vi "SP Update PF Indicator.vi"(5 "Parameters Measured":T9[](array[typedef]) {"Channel" min=1 max=99 step=1; "Parameter"."Stimulus Port" min=1 step=1; "Parameter"."Response Port" min=1 step=1}, 6 "References":T12, 7 "Pass? (f)":bool, 8 "Wait? (f)":bool, 9 "Filter Parameter":refnum<vi>, 10 "Limit Results":T1[](array[typedef]) {"Parameter"."Stimulus Port" min=1 step=1; "Parameter"."Response Port" min=1 step=1}, 11 "error in (no error)":errorcluster) -> (1 "Status Text":string, 3 "error out":errorcluster)   [LabVIEW 2011]
uses:
  TypeDefs/SP Parameter to Measure.ctl
  TypeDefs/SP Parameter.ctl
  TypeDefs/SP Calibration State.ctl
  TypeDefs/SP Measurement Format.ctl
  TypeDefs/SP Limit Results.ctl
  TypeDefs/SP Bandwidth Limit Results.ctl
  TypeDefs/SP Frequency Units.ctl
  TypeDefs/SP Ripple Limit Results.ctl
  TypeDefs/SP Format.ctl
  TypeDefs/SP Attenuation Limit Results.ctl
  TypeDefs/SP Skirt Limit Results.ctl
  <vilib>/Utility/miscctls.llb/LVRowAndColumnTypeDef.ctl
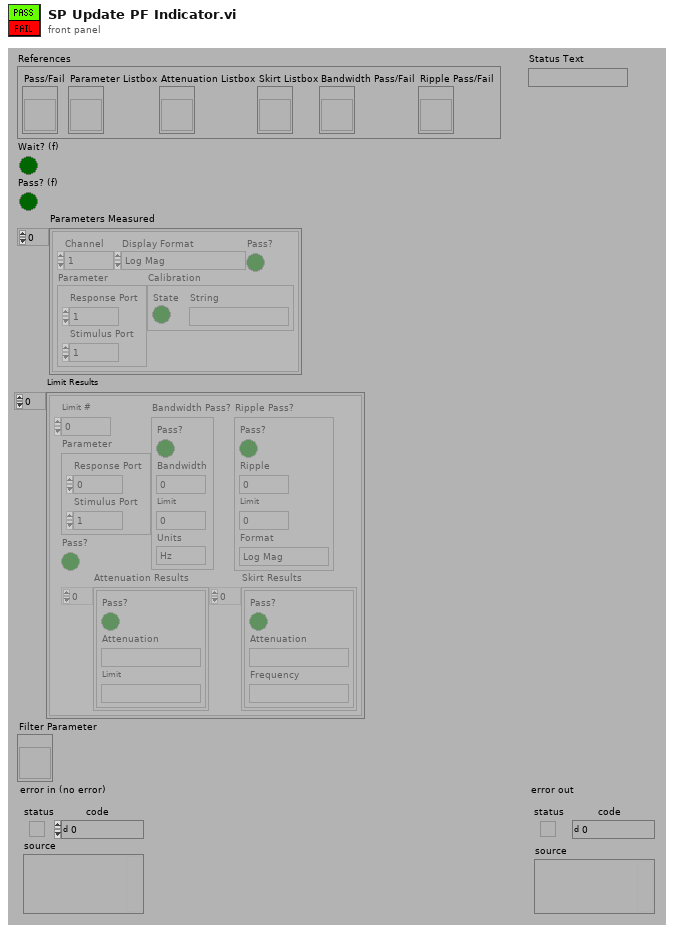
[diagram p1: front panel]
types:
  T1 = typedef "SP Limit Results.ctl" = cluster{"Limit #":i8, "Parameter":T2, "Bandwidth Pass?":T3, "Ripple Pass?":T5, "Attenuation Results":T7[], "Skirt Results":T8[], "Pass?":bool}
  T2 = typedef "SP Parameter.ctl" = cluster{"Stimulus Port":i8, "Response Port":i8}
  T3 = typedef "SP Bandwidth Limit Results.ctl" = cluster{"Pass?":bool, "Bandwidth":dbl, "Limit":dbl, "Units":T4}
  T4 = typedef "SP Frequency Units.ctl" = enum16{"Hz", "kHz", "MHz", "GHz", "Points"}
  T5 = typedef "SP Ripple Limit Results.ctl" = cluster{"Pass?":bool, "Ripple":dbl, "Limit":dbl, "Format":T6}
  T6 = typedef "SP Format.ctl" = enum16{"Log Mag", "Lin Mag", "SWR", "Phase", "Expanded Phase", "Delay", "Insertion Loss", "Isolation", "Return Loss"}
  T7 = typedef "SP Attenuation Limit Results.ctl" = cluster{"Pass?":bool, "Attenuation":string, "Limit":string}
  T8 = typedef "SP Skirt Limit Results.ctl" = cluster{"Pass?":bool, "Attenuation":string, "Frequency":string}
  T9 = typedef "SP Parameter to Measure.ctl" = cluster{"Channel":i8, "Parameter":T2, "Calibration":T10, "Display Format":T11, "Pass?":bool}
  T10 = typedef "SP Calibration State.ctl" = cluster{"State":bool, "String":string}
  T11 = typedef "SP Measurement Format.ctl" = enum32{"Log Mag", "Phase", "Delay", "Smith (R+jX)", "Polar (Re/Im)", "Linear Mag", "SWR", "Real", "Imaginary", "Smith (Lin/Phase)", "Smith (Log/Phase)", "Smith (Real/Imag)", "Smith (G+jB)", "Polar (Lin/Phase)", "Polar (Log/Phase)", "Expanded Phase", "Positive Phase", "Inverted Smith", "Unwrapped Phase", "Power Out", "Power In", "Linear Mag/Phase", "Log Mag/Phase", "Real/Imaginary"}
  T12 = cluster{"Pass/Fail":refnum<vi>, "Parameter Listbox":refnum<vi>, "Attenuation Listbox":refnum<vi>, "Skirt Listbox":refnum<vi>, "Bandwidth Pass/Fail":refnum<vi>, "Ripple Pass/Fail":refnum<vi>}
  T13 = typedef "LVRowAndColumnTypeDef.ctl" = cluster{"Row":i32, "Column":i32}
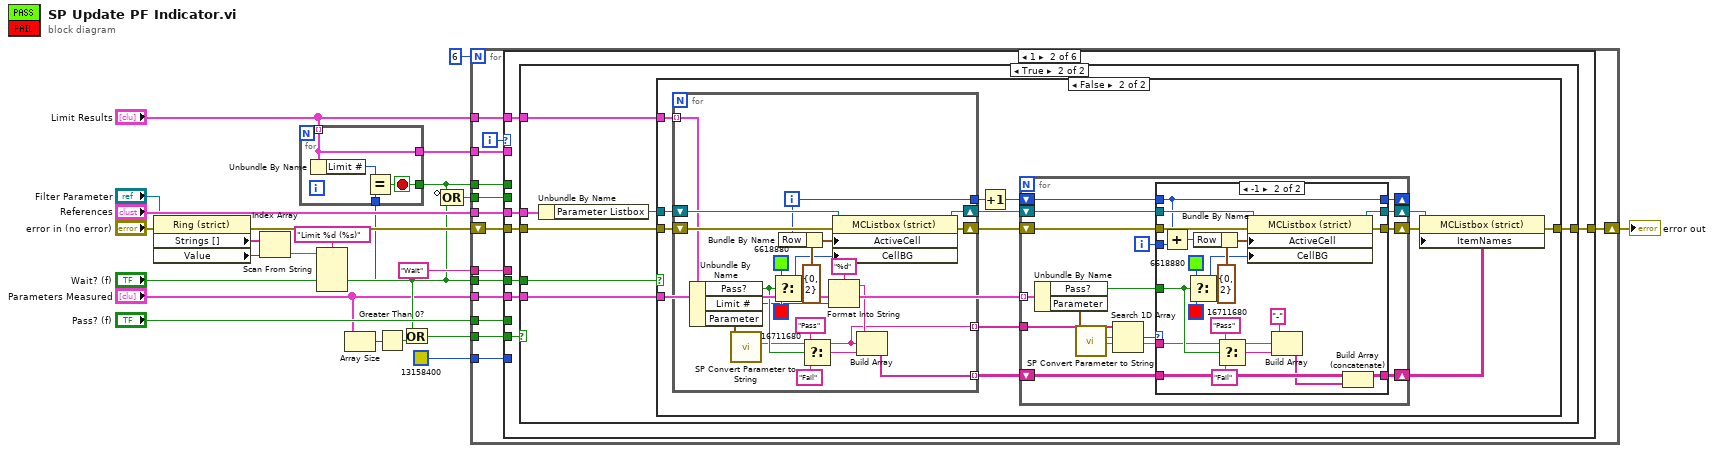
[diagram p0: block diagram]
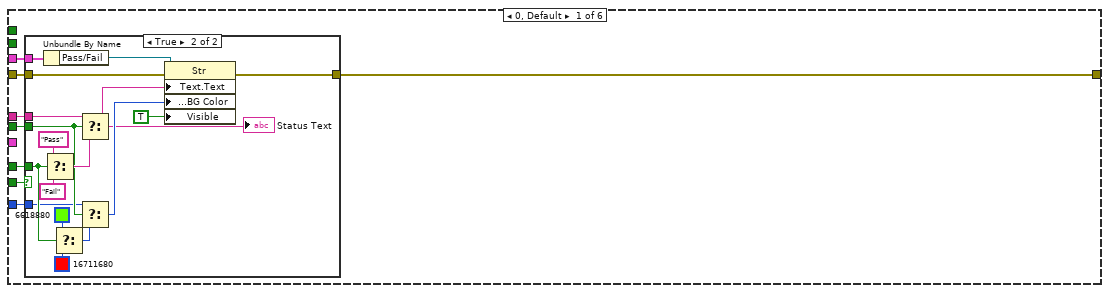
[diagram p2: hidden frame]
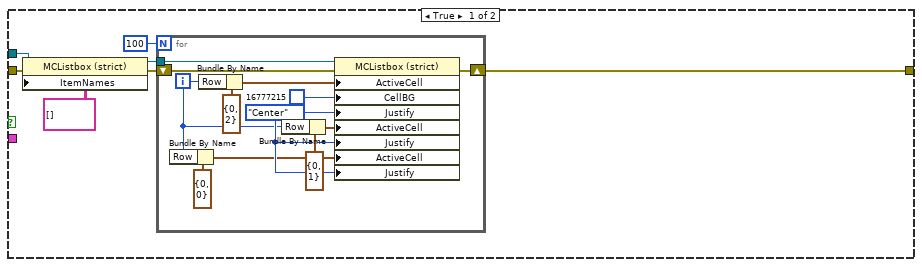
[diagram p5: hidden frame]
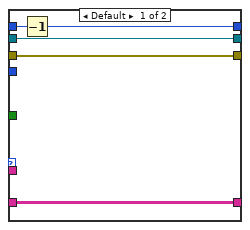
[diagram p6: hidden frame]
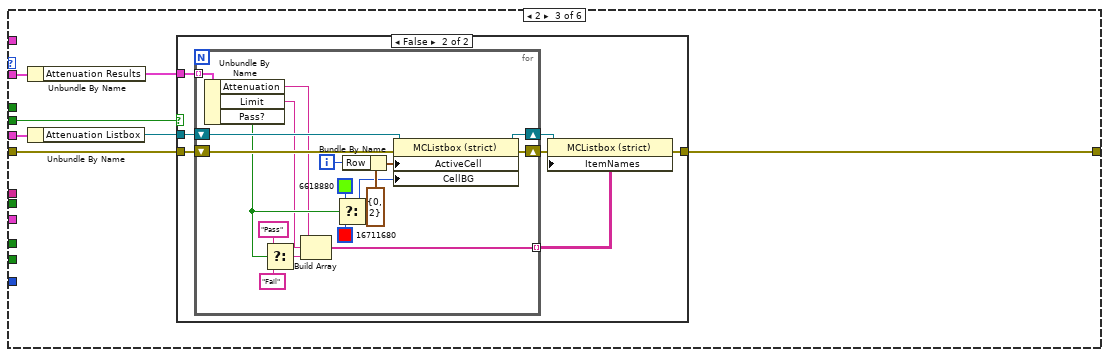
[diagram p7: hidden frame]
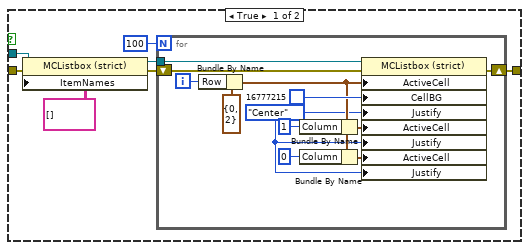
[diagram p8: hidden frame]
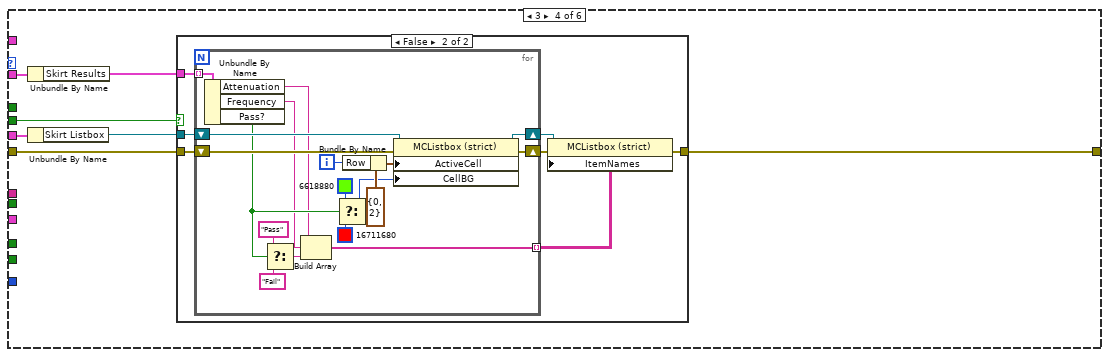
[diagram p9: hidden frame]
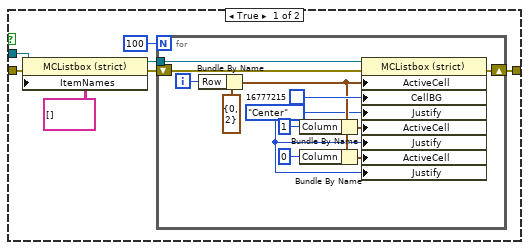
[diagram p10: hidden frame]
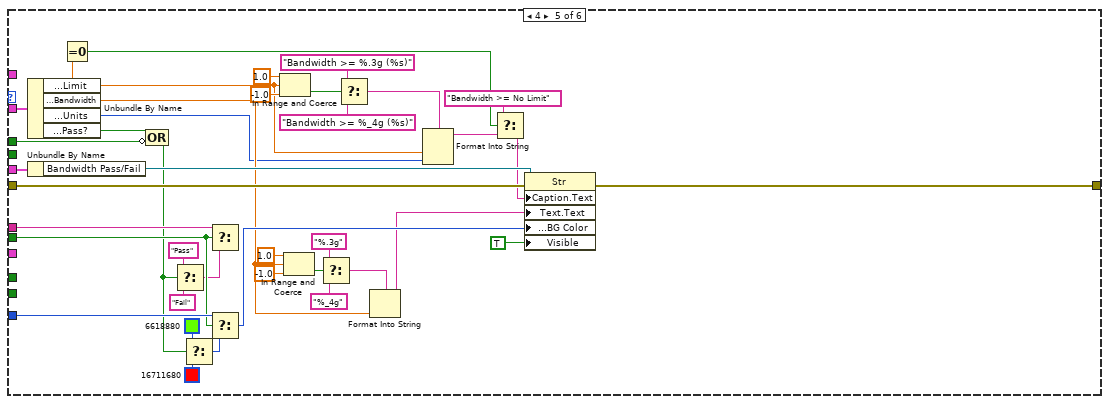
[diagram p11: hidden frame]
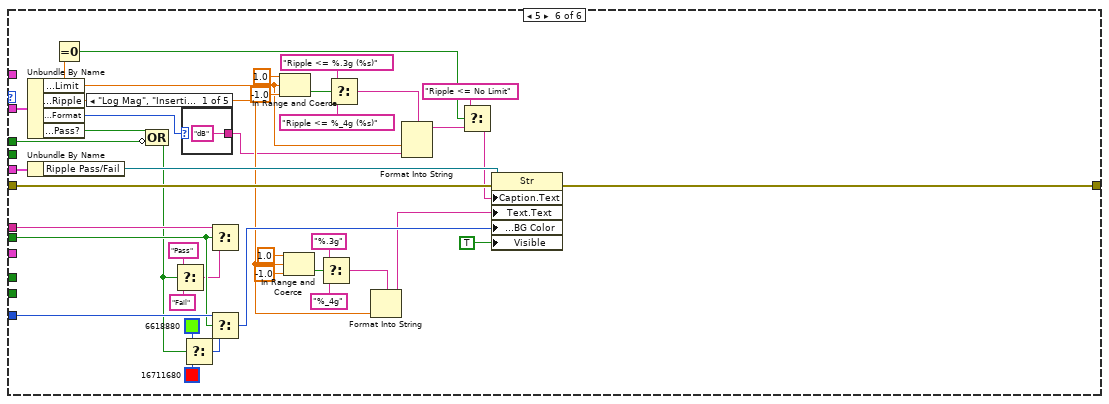
[diagram p12: hidden frame]
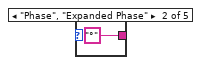
[diagram p13: hidden frame]
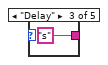
[diagram p14: hidden frame]
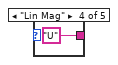
[diagram p15: hidden frame]
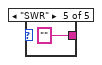
[diagram p16: hidden frame]
diagram:
  n1 = property class="Ring (strict)"(reference="Filter Parameter", error in="error in (no error)") -> (error out=w18:errorcluster, "Strings []"=w7:string[], "Value"=w6:i32)  [unwired: 1 out]
  n2 = Index Array(array=w7, index=w6) -> (element=w5:string)
  n3 = Scan From String(format string="Limit %d (%s)", input string=w5) -> (output 1=w3:i32)  [unwired: 2 in, 6 out]
  n4 = for {
    tunnel: "Limit Results" -> [w27] mode=indexing
    tunnel: [w27] -> w17
    tunnel: [w26] -> w10
    tunnel: w3 -> [w24]
    stop <- w26 stop-if-true
    n5 = Unbundle By Name(w27) -> ("Limit #"=w25:i8)
    n6 = Equal?(x=w25, y=w24) -> (x = y?=w26:bool)
  }
  n7 = Array Size(array="Parameters Measured") -> (size(s)=w13:i32)
  n8 = Greater Than 0?(x=w13) -> (x > 0?=w12:bool)
  n9 = Or(x="Wait? (f)", y=w12) -> (x .or. y?=w11:bool)
  n10 = Compound Arithmetic op=OR(invert w10, "Wait? (f)") -> (w8:bool)
  n11 = for {
    N: 6 -> [_]
    tunnel: "References" -> [w40]
    tunnel: "Wait? (f)" -> [w38]
    tunnel: "Parameters Measured" -> [w37]
    shift-right: [w39] -> w22
    shift-left: w18 -> [w41]
    tunnel: w17 -> [w35]
    tunnel: "Wait" -> [w34]
    tunnel: "Pass? (f)" -> [w33]
    tunnel: u32 13158400 -> [w32]
    tunnel: w11 -> [w31]
    tunnel: w10 -> [w30]
    tunnel: w8 -> [w29]
    tunnel: "Limit Results" -> [w28]
    i -> [w36]
    n12 = case shown="1" w36 {
      tunnel: w41 -> [w49 w74 w184 w233 w318 w358]
      tunnel: w40 -> [w47 w70 w182 w235 w316 w356]
      tunnel: [w48 w73 w183 w232 w317 w357] -> w39
      tunnel: w38 -> [w45 w72 _ _ w305 w345]
      tunnel: w37 -> [_ w71 _ _ _ _]
      tunnel: w35 -> [_ _ w180 w231 w309 w349]
      tunnel: w34 -> [w46 _ _ _ w306 w346]
      tunnel: w33 -> [w44 _ _ _ _ _]
      tunnel: w32 -> [w43 _ _ _ w307 w347]
      tunnel: w31 -> [w42 w69 _ _ _ _]
      tunnel: w30 -> [_ _ _ _ w302 w342]
      tunnel: w29 -> [_ _ w178 w229 _ _]
      tunnel: w28 -> [_ w68 _ _ _ _]
      frame 0, Default {
        n13 = case shown="True" w42 {
          tunnel: w49 -> [w50 w67]
          tunnel: [w50 w66] -> w48
          tunnel: w47 -> [_ w65]
          tunnel: w46 -> [_ w59]
          tunnel: w45 -> [_ w54]
          tunnel: w44 -> [_ w53]
          tunnel: w43 -> [_ w52]
          frame False {
          }
          frame True {
            n14 = Unbundle By Name(w65) -> ("Pass/Fail"=w64:refnum<vi>)
            n15 = Select(t="Pass", s=w53, f="Fail") -> (s? t:f=w60:string)
            n16 = Select(t=u32 6618880, s=w53, f=u32 16711680) -> (s? t:f=w58:u32)
            n17 = Select(t=w59, s=w54, f=w60) -> (s? t:f=w51:string)
            "Status Text" <- w51
            n18 = Select(t=w52, s=w54, f=w58) -> (s? t:f=w55:u32)
            n19 = property class="Str"(reference=w64, error in=w67, "Text.Text"=w51, "Text.Text Colors:BG Color"=w55, "Visible"=TRUE) -> (error out=w66:errorcluster)  [unwired: 1 out]
          }
        }
      }
      frame 1 {
        n20 = case shown="True" w69 {
          tunnel: w74 -> [w75 w82]
          tunnel: [w75 w81] -> w73
          tunnel: w72 -> [_ w80]
          tunnel: w71 -> [_ w79]
          tunnel: w70 -> [_ w78]
          tunnel: w68 -> [_ w76]
          frame False {
          }
          frame True {
            n21 = Unbundle By Name(w78) -> ("Parameter Listbox"=w77:refnum<vi>)
            n22 = case shown="False" w80 {
              tunnel: w82 -> [w84 w107]
              tunnel: w77 -> [w83 w108]
              tunnel: [w88 w115] -> w81
              tunnel: w79 -> [_ w113]
              tunnel: w76 -> [_ w114]
              frame True {
                n23 = property class="MCListbox (strict)"(reference=w83, error in=w84, "ItemNames"=string[][] [] ("Item Names")) -> (reference out=w86:refnum<vi>, error out=w87:errorcluster)
                n24 = for {
                  N: 100 -> [_]
                  shift-right: [w100] -> w88
                  shift-left: w87 -> [w101]
                  tunnel: w86 -> [w96]
                  i -> [w90]
                  w93 = enum16{"Left", "Center", "Right"}."Center" ("Active Cell:Cell Justification")
                  n25 = Bundle By Name(cluster=T13 {"Row"=0, "Column"=0} ("Active Cell:Active Cell"), "Row"=w90) -> (w92:T13)
                  n26 = Bundle By Name(cluster=T13 {"Row"=0, "Column"=2} ("Active Cell:Active Cell"), "Row"=w90) -> (w98:T13)
                  n27 = Bundle By Name(cluster=T13 {"Row"=0, "Column"=1} ("Active Cell:Active Cell"), "Row"=w90) -> (w94:T13)
                  n28 = property class="MCListbox (strict)"(reference=w96, error in=w101, "ActiveCell"=w98, "CellBG"=u32 16777215, "Justify"=w93, "ActiveCell"=w94, "Justify"=w93, "ActiveCell"=w92, "Justify"=w93) -> (error out=w100:errorcluster)  [unwired: 1 out]
                }
              }
              frame False {
                n29 = for {
                  shift-right: [w176] -> w110
                  shift-left: w107 -> [w177]
                  shift-right: [w169] -> w109
                  shift-left: w108 -> [w173]
                  tunnel: w114 -> [w164] mode=indexing
                  tunnel: [w159] -> w102 mode=indexing
                  tunnel: [w158] -> w105 mode=indexing
                  tunnel: [w157] -> w103
                  i -> [w157]
                  n30 = Unbundle By Name(w164) -> ("Pass?"=w166:bool, "Limit #"=w161:i8, "Parameter"=w162:T2)
                  n31 = call "SP Convert Parameter to String.vi"("Parameter"=w162) -> ("Parameter String"=w159:string)  [unwired: 10 out]
                  n32 = Select(t=u32 6618880, s=w166, f=u32 16711680) -> (s? t:f=w170:u32)
                  n33 = Bundle By Name(cluster=T13 {"Row"=0, "Column"=2} ("Active Cell:Active Cell"), "Row"=w157) -> (w174:T13)
                  n34 = Select(t="Pass", s=w166, f="Fail") -> (s? t:f=w165:string)
                  n35 = Format Into String(format string="%d", w161) -> (resulting string=w160:string)  [unwired: 2 in, 1 out]
                  n36 = property class="MCListbox (strict)"(reference=w173, error in=w177, "ActiveCell"=w174, "CellBG"=w170) -> (reference out=w169:refnum<vi>, error out=w176:errorcluster)
                  n37 = Build Array(w160, w159, w165) -> (w158:string[])
                }
                n38 = Increment(x=w103) -> (x+1=w106:i32)
                n39 = for {
                  shift-right: [w129] -> w111
                  shift-left: w110 -> [w130]
                  shift-right: [w127] -> w112
                  shift-left: w109 -> [w128]
                  tunnel: w113 -> [w125] mode=indexing
                  shift-right: [w117] -> w104
                  shift-left: w105 -> [w118]
                  tunnel: w102 -> [w121]
                  shift-right: [w116] -> _
                  shift-left: w106 -> [w123]
                  i -> [w122]
                  n40 = Unbundle By Name(w125) -> ("Pass?"=w126:bool, "Parameter"=w124:T2)
                  n41 = call "SP Convert Parameter to String.vi"("Parameter"=w124) -> ("Parameter String"=w119:string)  [unwired: 10 out]
                  n42 = Search 1D Array(1D array=w121, element=w119) -> (index of element=w120:i32)  [unwired: 1 out]
                  n43 = case shown="-1" w120 {
                    tunnel: w130 -> [w134 w156]
                    tunnel: [w134 w155] -> w129
                    tunnel: w128 -> [w135 w152]
                    tunnel: [w135 w148] -> w127
                    tunnel: w126 -> [_ w145]
                    tunnel: w119 -> [_ w143]
                    tunnel: w123 -> [w132 w136]
                    tunnel: w122 -> [_ w140]
                    tunnel: w118 -> [w133 w139]
                    tunnel: [w133 w137] -> w117
                    tunnel: [w131 w136] -> w116
                    frame Default {
                      n44 = Decrement(x=w132) -> (x-1=w131:i32)
                    }
                    frame -1 {
                      n45 = Add(x=w136, y=w140) -> (x+y=w141:i32)
                      n46 = Select(t=u32 6618880, s=w145, f=u32 16711680) -> (s? t:f=w149:u32)
                      n47 = Bundle By Name(cluster=T13 {"Row"=0, "Column"=2} ("Active Cell:Active Cell"), "Row"=w141) -> (w153:T13)
                      n48 = Select(t="Pass", s=w145, f="Fail") -> (s? t:f=w144:string)
                      n49 = property class="MCListbox (strict)"(reference=w152, error in=w156, "ActiveCell"=w153, "CellBG"=w149) -> (reference out=w148:refnum<vi>, error out=w155:errorcluster)
                      n50 = Build Array("-" ("format string"), w143, w144) -> (w138:string[])
                      n51 = Build Array (concatenate)(w139, w138) -> (w137:string[][])
                    }
                  }
                }
                n52 = property class="MCListbox (strict)"(reference=w112, error in=w111, "ItemNames"=w104) -> (error out=w115:errorcluster)  [unwired: 1 out]
              }
            }
          }
        }
      }
      frame 2 {
        n53 = Unbundle By Name(w180) -> ("Attenuation Results"=w179:T7[])
        n54 = Unbundle By Name(w182) -> ("Attenuation Listbox"=w181:refnum<vi>)
        n55 = case shown="False" w178 {
          tunnel: w184 -> [w186 w206]
          tunnel: w181 -> [w185 w205]
          tunnel: [w190 w208] -> w183
          tunnel: w179 -> [_ w204]
          frame True {
            n56 = property class="MCListbox (strict)"(reference=w185, error in=w186, "ItemNames"=string[][] [] ("Item Names")) -> (reference out=w188:refnum<vi>, error out=w189:errorcluster)
            n57 = for {
              N: 100 -> [_]
              shift-right: [w202] -> w190
              shift-left: w189 -> [w203]
              tunnel: w188 -> [w199]
              i -> [w197]
              w192 = enum16{"Left", "Center", "Right"}."Center" ("Active Cell:Cell Justification")
              n58 = Bundle By Name(cluster=T13 {"Row"=0, "Column"=2} ("Active Cell:Active Cell"), "Row"=w197) -> (w194:T13)
              n59 = Bundle By Name(cluster=w194, "Column"=1) -> (w198:T13)
              n60 = Bundle By Name(cluster=w194, "Column"=0) -> (w193:T13)
              n61 = property class="MCListbox (strict)"(reference=w199, error in=w203, "ActiveCell"=w194, "CellBG"=u32 16777215, "Justify"=w192, "ActiveCell"=w198, "Justify"=w192, "ActiveCell"=w193, "Justify"=w192) -> (error out=w202:errorcluster)  [unwired: 1 out]
            }
          }
          frame False {
            n62 = for {
              shift-right: [w227] -> w210
              shift-left: w206 -> [w228]
              shift-right: [w219] -> w209
              shift-left: w205 -> [w223]
              tunnel: [w215] -> w207 mode=indexing
              tunnel: w204 -> [w214] mode=indexing
              i -> [w225]
              n63 = Unbundle By Name(w214) -> ("Attenuation"=w212:string, "Limit"=w211:string, "Pass?"=w213:bool)
              n64 = Select(t="Pass", s=w213, f="Fail") -> (s? t:f=w216:string)
              n65 = Build Array(w212, w211, w216) -> (w215:string[])
              n66 = Select(t=u32 6618880, s=w213, f=u32 16711680) -> (s? t:f=w220:u32)
              n67 = Bundle By Name(cluster=T13 {"Row"=0, "Column"=2} ("Active Cell:Active Cell"), "Row"=w225) -> (w224:T13)
              n68 = property class="MCListbox (strict)"(reference=w223, error in=w228, "ActiveCell"=w224, "CellBG"=w220) -> (reference out=w219:refnum<vi>, error out=w227:errorcluster)
            }
            n69 = property class="MCListbox (strict)"(reference=w209, error in=w210, "ItemNames"=w207) -> (error out=w208:errorcluster)  [unwired: 1 out]
          }
        }
      }
      frame 3 {
        n70 = Unbundle By Name(w231) -> ("Skirt Results"=w230:T8[])
        n71 = Unbundle By Name(w235) -> ("Skirt Listbox"=w234:refnum<vi>)
        n72 = case shown="False" w229 {
          tunnel: w233 -> [w241 w257]
          tunnel: w234 -> [w240 w256]
          tunnel: [w236 w259] -> w232
          tunnel: w230 -> [_ w255]
          frame True {
            n73 = property class="MCListbox (strict)"(reference=w240, error in=w241, "ItemNames"=string[][] [] ("Item Names")) -> (reference out=w238:refnum<vi>, error out=w239:errorcluster)
            n74 = for {
              N: 100 -> [_]
              shift-right: [w253] -> w236
              shift-left: w239 -> [w254]
              tunnel: w238 -> [w250]
              i -> [w248]
              w243 = enum16{"Left", "Center", "Right"}."Center" ("Active Cell:Cell Justification")
              n75 = Bundle By Name(cluster=T13 {"Row"=0, "Column"=2} ("Active Cell:Active Cell"), "Row"=w248) -> (w245:T13)
              n76 = Bundle By Name(cluster=w245, "Column"=1) -> (w249:T13)
              n77 = Bundle By Name(cluster=w245, "Column"=0) -> (w244:T13)
              n78 = property class="MCListbox (strict)"(reference=w250, error in=w254, "ActiveCell"=w245, "CellBG"=u32 16777215, "Justify"=w243, "ActiveCell"=w249, "Justify"=w243, "ActiveCell"=w244, "Justify"=w243) -> (error out=w253:errorcluster)  [unwired: 1 out]
            }
          }
          frame False {
            n79 = for {
              shift-right: [w278] -> w261
              shift-left: w257 -> [w279]
              shift-right: [w270] -> w260
              shift-left: w256 -> [w274]
              tunnel: [w266] -> w258 mode=indexing
              tunnel: w255 -> [w265] mode=indexing
              i -> [w276]
              n80 = Unbundle By Name(w265) -> ("Attenuation"=w263:string, "Frequency"=w262:string, "Pass?"=w264:bool)
              n81 = Select(t="Pass", s=w264, f="Fail") -> (s? t:f=w267:string)
              n82 = Build Array(w263, w262, w267) -> (w266:string[])
              n83 = Select(t=u32 6618880, s=w264, f=u32 16711680) -> (s? t:f=w271:u32)
              n84 = Bundle By Name(cluster=T13 {"Row"=0, "Column"=2} ("Active Cell:Active Cell"), "Row"=w276) -> (w275:T13)
              n85 = property class="MCListbox (strict)"(reference=w274, error in=w279, "ActiveCell"=w275, "CellBG"=w271) -> (reference out=w270:refnum<vi>, error out=w278:errorcluster)
            }
            n86 = property class="MCListbox (strict)"(reference=w260, error in=w261, "ItemNames"=w258) -> (error out=w259:errorcluster)  [unwired: 1 out]
          }
        }
      }
      frame 4 {
        n87 = Unbundle By Name(w309) -> ("Bandwidth Pass?.Limit"=w284:dbl, "Bandwidth Pass?.Bandwidth"=w286:dbl, "Bandwidth Pass?.Units"=w285:T4, "Bandwidth Pass?.Pass?"=w301:bool)
        n88 = Unbundle By Name(w316) -> ("Bandwidth Pass/Fail"=w315:refnum<vi>)
        n89 = Equal To 0?(x=w284) -> (x = 0?=w280:bool)
        n90 = Compound Arithmetic op=OR(w301, invert w302) -> (w300:bool)
        n91 = Select(t="Pass", s=w300, f="Fail") -> (s? t:f=w304:string)
        n92 = Select(t=u32 6618880, s=w300, f=u32 16711680) -> (s? t:f=w308:u32)
        n93 = Select(t=w306, s=w305, f=w304) -> ()  [unwired: 1 out]
        n94 = Select(t=w307, s=w305, f=w308) -> (s? t:f=w303:u32)
        n95 = In Range and Coerce(upper limit=1.0, x=w284, lower limit=-1.0) -> (In Range?=w296:bool)  [unwired: 1 out]
        n96 = In Range and Coerce(upper limit=1.0, x=w286, lower limit=-1.0) -> (In Range?=w292:bool)  [unwired: 1 out]
        n97 = Select(t="%.3g" ("format string"), s=w292, f="%_4g" ("format string")) -> (s? t:f=w288:string)
        n98 = Select(t="Bandwidth >= %.3g (%s)" ("format string"), s=w296, f="Bandwidth >= %_4g (%s)" ("format string")) -> (s? t:f=w294:string)
        n99 = Format Into String(format string=w288, w286) -> (resulting string=w287:string)  [unwired: 2 in, 1 out]
        n100 = Format Into String(format string=w294, w284, w285) -> (resulting string=w283:string)  [unwired: 2 in, 1 out]
        n101 = Select(t="Bandwidth >= No Limit" ("format string"), s=w280, f=w283) -> (s? t:f=w281:string)
        n102 = property class="Str"(reference=w315, error in=w318, "Caption.Text"=w281, "Text.Text"=w287, "Text.Text Colors:BG Color"=w303, "Visible"=TRUE) -> (error out=w317:errorcluster)  [unwired: 1 out]
      }
      frame 5 {
        n103 = Unbundle By Name(w349) -> ("Ripple Pass?.Limit"=w322:dbl, "Ripple Pass?.Ripple"=w326:dbl, "Ripple Pass?.Format"=w325:T6, "Ripple Pass?.Pass?"=w341:bool)
        n104 = Unbundle By Name(w356) -> ("Ripple Pass/Fail"=w355:refnum<vi>)
        n105 = Equal To 0?(x=w322) -> (x = 0?=w321:bool)
        n106 = Compound Arithmetic op=OR(w341, invert w342) -> (w340:bool)
        n107 = Select(t="Pass", s=w340, f="Fail") -> (s? t:f=w344:string)
        n108 = case shown="\"Log Mag\", \"Insertion Loss\"..\"Return Loss\", Default" w325 {
          tunnel: ["dB" "°" "s" "U" ""] -> w324
          frame "Log Mag", "Insertion Loss".."Return Loss", Default {
          }
          frame "Phase", "Expanded Phase" {
          }
          frame "Delay" {
          }
          frame "Lin Mag" {
          }
          frame "SWR" {
          }
        }
        n109 = Select(t=u32 6618880, s=w340, f=u32 16711680) -> (s? t:f=w348:u32)
        n110 = Select(t=w346, s=w345, f=w344) -> ()  [unwired: 1 out]
        n111 = Select(t=w347, s=w345, f=w348) -> (s? t:f=w343:u32)
        n112 = In Range and Coerce(upper limit=1.0, x=w322, lower limit=-1.0) -> (In Range?=w336:bool)  [unwired: 1 out]
        n113 = In Range and Coerce(upper limit=1.0, x=w326, lower limit=-1.0) -> (In Range?=w332:bool)  [unwired: 1 out]
        n114 = Select(t="%.3g" ("format string"), s=w332, f="%_4g" ("format string")) -> (s? t:f=w328:string)
        n115 = Select(t="Ripple <= %.3g (%s)" ("format string"), s=w336, f="Ripple <= %_4g (%s)" ("format string")) -> (s? t:f=w334:string)
        n116 = Format Into String(format string=w328, w326) -> (resulting string=w327:string)  [unwired: 2 in, 1 out]
        n117 = Format Into String(format string=w334, w322, w324) -> (resulting string=w320:string)  [unwired: 2 in, 1 out]
        n118 = Select(t="Ripple <= No Limit" ("format string"), s=w321, f=w320) -> (s? t:f=w319:string)
        n119 = property class="Str"(reference=w355, error in=w358, "Caption.Text"=w319, "Text.Text"=w327, "Text.Text Colors:BG Color"=w343, "Visible"=TRUE) -> (error out=w357:errorcluster)  [unwired: 1 out]
      }
    }
  }
  "error out" <- w22
